vi "Set Setup Display Zoom to Fit Image.vi"(8 "error in (no error)":errorcluster, 10 "Size":T2, 11 "UI in":refnum<class "UI.lvclass">) -> (0 "error out":errorcluster, 2 "Offset":T1)   [LabVIEW 2020, in "AR Example.lvlib" / "UI.lvclass"]
uses:
  UI.lvclass
  UI.lvclass/UI.ctl
  g_ar_toolkit.common/Image Size (Integer).ctl
  g_ar_toolkit.image/Image Draw Offset.ctl
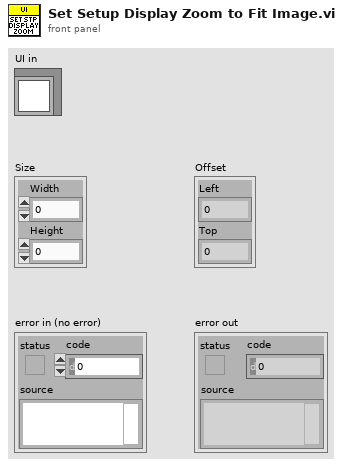
[diagram p1: front panel]
types:
  T1 = typedef "g_ar_toolkit.image.lvlib/Image Draw Offset.ctl" = cluster{"Left":i16, "Top":i16}
  T2 = typedef "g_ar_toolkit.common.lvlib/Image Size (Integer).ctl" = cluster{"Width":u16, "Height":u16}
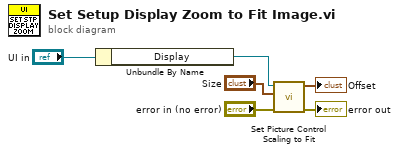
[diagram p0: block diagram]
diagram:
  n1 = Unbundle By Name("UI in") -> ("Display"=w5:refnum<vi>)
  n2 = call "Set Picture Control Scaling to Fit.vi"("error in (no error)"="error in (no error)", "Image Size"="Size", "Picture in"=w5) -> ("error out"=→"error out":errorcluster, "Image Draw Offset"=→"Offset":T1)  [unwired: 7 in]
